vi "Polynomial Roots.vi"   [LabVIEW 2014, in "NI_AALPro.lvlib"]
doc: "Finds the roots of polynomial <B>P(x)</B>. This VI removes leading coefficients of the polynomial that are equal to zero. Wire data to the <B>P(x)</B> input to determine the polymorphic instance to use or manually select the instance."
uses:
  NI_AALPro.lvlib
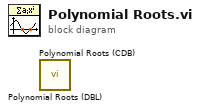
[diagram p0: block diagram]
diagram:
  n1 = call "Polynomial Roots (DBL).vi"() -> ()  [unwired: 10 in, 2 out]
  n2 = call "Polynomial Roots (CDB).vi"() -> ()  [unwired: 10 in, 2 out]
